vi "FRCts20_WebMethods_ErrorHandler.vi"(8 "error in":errorcluster, 11 "LabVIEW Web Service Request":refnum<class "Web Request.lvclass">) -> (0 "error out":errorcluster, 3 "LabVIEW Web Service Request":refnum<class "Web Request.lvclass">)   [LabVIEW 2014, in "FRCts20_WebMethods.lvlib"]
doc: "This subVI writes a HTTP response if an error occurs in the web service and the application ini file has a TRUE debug flag.\n\nThe code and source are converted to string and written to HTTP Request."
uses:
  FRCts20_WebMethods.lvlib
  <vilib>/wsapi/Web Request.lvclass
  Backend/source/VI Source/INI_Accessor/FRCts20_Backend_INI Controller.lvclass
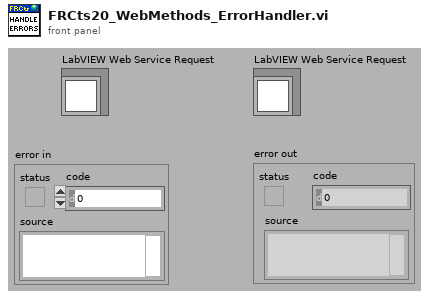
[diagram p1: front panel]
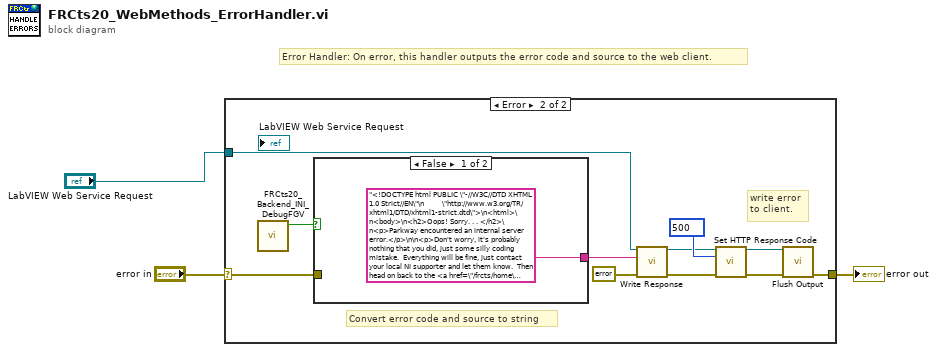
[diagram p0: block diagram]
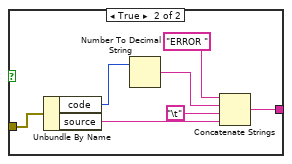
[diagram p3: hidden frame]
diagram:
  # "Error Handler: On error, this handler outputs the error code and source to the web client."
  n1 = case shown="Error" "error in" {
    selector: "error in" -> [w4 w11]
    tunnel: [w4 w15] -> w3
    tunnel: "LabVIEW Web Service Request" -> [_ w5]
    frame No Error {
    }
    frame Error {
      w13 = 500 items=["100"=100, "101"=101, "200"=200, "201"=201, "202"=202, "203"=203, "204"=204, "205"=205, "206"=206, "300"=300, "301"=301, "302"=302, "303"=303, "304"=304, "305"=305, "306"=306, "307"=307, "400"=400, "401"=401, "402"=402, "403"=403, "404"=404, "405"=405, "406"=406, "407"=407, "408"=408, "409"=409, "410"=410, "411"=411, "412"=412, "413"=413, "414"=414, "415"=415, "416"=416, "417"=417, "500"=500, "501"=501, "502"=502, "503"=503, "504"=504, "505"=505] ("response code (200)")
      # "write error \nto client."
      # "Convert error code and source to string"
      n2 = call "FRCts20_Backend_INI_DebugFGV.vi"() -> ("Value out"=w12:bool)  [unwired: 11 in]
      n3 = case shown="False" w12 {
        tunnel: w11 -> [_ w18]
        tunnel: ["<!DOCTYPE html PUBLIC \"-//W3C//DTD XHTML 1.0 Strict//EN\"\n         \"http://www.w3.org/TR/xhtml1/DTD/xhtml1-strict.dtd\">\n<html>\n<body>\n<h2>Oops! Sorry. . . </h2>\n<p>Parkway encountered an internal server error.</p>\n\n<p>Don't worry, it's probably nothing that you did, just some silly coding mistake.  Everything will be fine, just contact your local NI supporter and let them know.  Then head on back to the <a href=\"/frcts/home\">home page</a> and try again! </p>\n\n<img src=\"http://www.ni.com/images/homepage/us/logo.gif\" alt=\"National Instruments logo\">\n<img src=\"http://www.usfirst.org/sites/all/themes/first_core/logo.png\" alt=\"FIRST logo\">\n</body>\n</html>" w17] -> w8
        frame False {
        }
        frame True {
          n4 = Unbundle By Name(w18) -> ("code"=w23:i32, "source"=w20:string)
          n5 = Number To Decimal String(number=w23) -> (decimal integer string=w22:string)  [unwired: 1 in]
          n6 = Concatenate Strings("ERROR " ("string"), w22, "\t", w20) -> (w17:string)
        }
      }
      n7 = call <vilib>:"Write Response.vi"("LabVIEW Web Service Request"=w5, "response string"=w8, "error in (no error)"=errorcluster {"status"=FALSE, "code"=0, "source"=""}) -> ("LabVIEW Web Service Request out"=w6:refnum<class "Web Request.lvclass">, "error out"=w9:errorcluster)  [unwired: 11 in]
      n8 = call <vilib>:"Set HTTP Response Code.vi"("LabVIEW Web Service Request"=w6, "response code (200)"=w13, "error in (no error)"=w9) -> ("LabVIEW Web Service Request out"=w7:refnum<class "Web Request.lvclass">, "error out"=w14:errorcluster)  [unwired: 11 in]
      n9 = call <vilib>:"Flush Output.vi"("LabVIEW Web Service Request"=w7, "error in (no error)"=w14) -> ("error out"=w15:errorcluster)  [unwired: 12 in, 1 out]
    }
  }
  "error out" <- w3
